vi "retrieveCommonCfg.vi"(8 "error in (no error)":errorcluster, 10 "dataName":string, 11 "ConfigurationFileReader in":refnum<class "ConfigurationFileReader.lvclass">) -> (0 "error out":errorcluster, 2 "dataValueFromFile":string, 3 "ConfigurationFileReader out":refnum<class "ConfigurationFileReader.lvclass">)   [LabVIEW 2016, in "Settings.lvlib" / "ConfigurationFileReader.lvclass"]
uses:
  ConfigurationFileReader.lvclass
  <vilib>/Utility/xml.llb/Read From XML File(string).vi
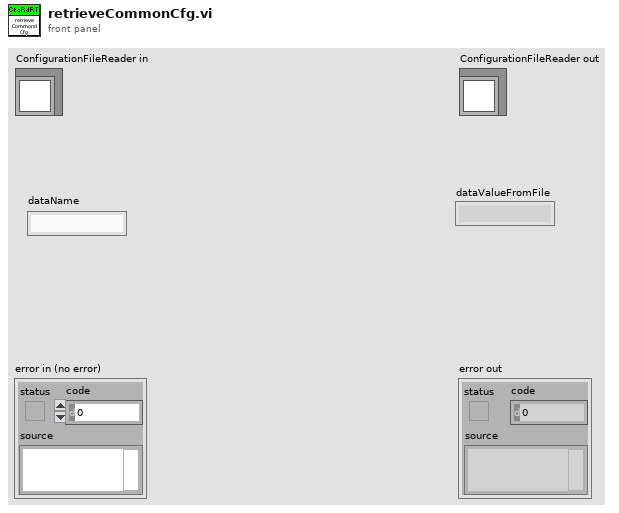
[diagram p1: front panel]
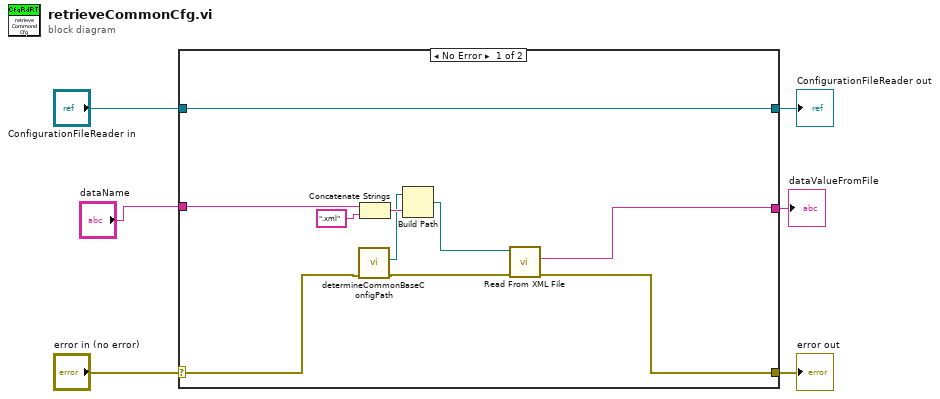
[diagram p0: block diagram]
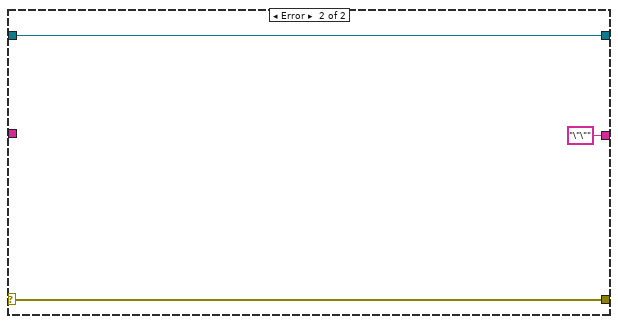
[diagram p2: hidden frame]
diagram:
  n1 = case shown="No Error" "error in (no error)" {
    selector: "error in (no error)" -> [w8 w19]
    tunnel: [w11 w19] -> w5
    tunnel: [w16 w18] -> w3
    tunnel: "ConfigurationFileReader in" -> [w16 w18]
    tunnel: "dataName" -> [w12 _]
    tunnel: [w10 "\"\"" ("XML Elements")] -> w1
    frame No Error {
      n2 = call "determineCommonBaseConfigPath.vi"("error in (no error)"=w8) -> ("error out"=w9:errorcluster, "ConfigurationPath"=w7:path)  [unwired: 8 in, 1 out]
      n3 = Concatenate Strings(w12, ".xml" ("string")) -> (w13:string)
      n4 = Build Path(base path=w7, name or relative path=w13) -> (appended path=w14:path)
      n5 = call-poly <vilib>:"Read From XML File.vi"("error in (no error)"=w9, "XML File Path"=w14) -> ("error out"=w11:errorcluster, "XML Elements"=w10:string)  [unwired: 7 in, 1 out]
    }
    frame Error {
    }
  }
  "error out" <- w5
  "ConfigurationFileReader out" <- w3
  "dataValueFromFile" <- w1
